vi "初始化选择第一个状态.vi"(0 "测试项目队列输入":refnum<queue>) -> (1 "切换卡片":T2(ring)=enum."指令测试", 2 "当前状态":T1)   [LabVIEW 2015]
panel:
  out "测试项目队列输出":refnum<queue>
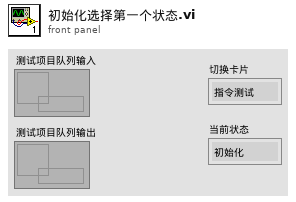
[diagram p1: front panel]
types:
  T1 = typedef "状态机状态.ctl" = enum16{"初始化", "等待按键", "串口操作", "检索模块", "网络测试", "测试项目", "模块参数配置", "指令测试", "数据测试", "特殊功能测试", "心跳包测试", "升级测试", "中心切换测试", "计算测试耗时", "生成报告", "提示消息", "退出"}
  T2 = enum32{"主界面", "初始化配置", "指令测试", "数据测试", "特殊功能测试", "心跳包测试", "升级测试", "中心切换测试", "生成报告"}
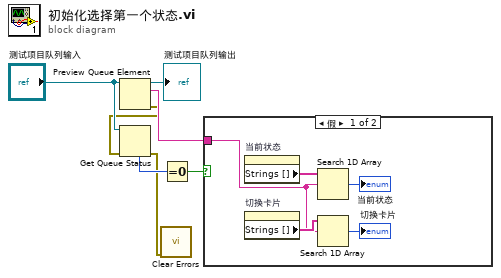
[diagram p0: block diagram]
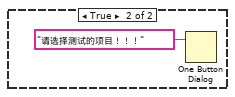
[diagram p2: hidden frame]
diagram:
  n1 = Preview Queue Element(queue="测试项目队列输入") -> (queue out=→"测试项目队列输出":refnum<queue>, element=w3:string, error out=w1:errorcluster)  [unwired: 2 in, 1 out]
  n2 = Get Queue Status(queue="测试项目队列输入", error in (no error)=w1) -> (error out=w2:errorcluster, # elements in queue=w4:i32)  [unwired: 1 in, 6 out]
  n3 = call <vilib>:"Clear Errors.vi"("error in (no error)"=w2) -> ()  [unwired: 5 in, 2 out]
  n4 = Equal To 0?(x=w4) -> (x = 0?=w7:bool)
  n5 = case shown="假" w7 {
    tunnel: w3 -> [w8 _]
    frame False {
      n6 = property on="当前状态" class="Enum (严格)"() -> ("Strings []"=w9:string[])  [unwired: 2 in, 2 out]
      n7 = property on="切换卡片" class="Enum (严格)"() -> ("Strings []"=w11:string[])  [unwired: 2 in, 2 out]
      n8 = Search 1D Array(1D array=w9, element=w8) -> (index of element=→"当前状态":i32)  [unwired: 1 in]
      n9 = Search 1D Array(1D array=w11, element=w8) -> (index of element=→"切换卡片":i32)  [unwired: 1 in]
    }
    frame True {
      n10 = One Button Dialog(message="请选择测试的项目！！！" ("消息")) -> ()  [unwired: 1 in, 1 out]
    }
  }
